vi "FindStats.vi"(7 "Actor":refnum<class "Actor.lvclass">) -> (3 "Stats":T1)   [LabVIEW 2020, in "jettl.lvlib" / "Actor.lvclass"]
uses:
  Actor.lvclass
  Msg/Msg.lvclass
  MsgSet.ctl
  jettl.lvlib
  Stats.ctl
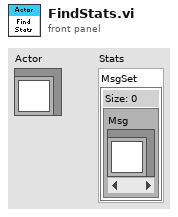
[diagram p1: front panel]
types:
  T1 = typedef "jettl.lvlib/Stats.ctl" = cluster{"MsgSet":T2}
  T2 = typedef "jettl.lvlib/MsgSet.ctl" = set{refnum<class "Msg.lvclass">}
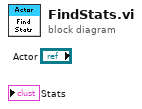
[diagram p0: block diagram]
diagram:
